vi "Start Module.vi"(6 "Show Main VI Diagram on Init (F)":bool, 8 "error in":errorcluster, 9 "Init Module ID":bool, 10 "Number of socket":i32, 11 "Run as Singleton? (F)":bool) -> (0 "error out":errorcluster, 1 "Wait for Event Sync?":bool, 2 "Test Unit Broadcast Events":T1, 3 "Module ID":i32)   [LabVIEW 2025, in "Test Unit.lvlib"]
doc: "Launches an instance of the module Main VI. After calling this VI, you can optionally register for broadcast events from the module by wiring the broadcast events output of this VI to a <b>Register For Events</b> function. \n\nAfter the optional Register For Events function call, you should always call the <b>Synchronize Module Events.vi</b> for this module with the 'Wait for Event Sync?' output of this VI to the corresponding input of the Synchronize Module Events.vi. \n\nTo see an example of the proper wiring pattern, see the \"Run New Module: Value Change\" event frame in the API Tester VI for this module.\n_____\nBased on DQMH Project Template 7.0.1.1316."
uses:
  Test Unit.lvlib
  Broadcast Events--cluster.ctl
  Did Init Argument--cluster.ctl
  Status Updated Argument--cluster.ctl
  Error Reported Argument--cluster.ctl
  Stop Argument--cluster.ctl
  Get Module Execution Status Argument--cluster.ctl
  Module Running State--enum.ctl
  <vilib>/Delacor/Delacor QMH/Libraries/Cloneable Module Admin_class/Delacor_lib_QMH_Cloneable Module Admin.lvclass
  C:/Program Files (x86)/National Instruments/LabVIEW 2025/vi.lib/Delacor/Delacor QMH/Libraries/Module Admin_class/Delacor_lib_QMH_Module Admin.lvclass
  VI Reference Management/Main VI Type--strict_vi_ref.ctl
  <vilib>/Delacor/Delacor QMH/Libraries/Cloneable Module Admin_class/Delacor_lib_QMH_Cloneable Module Admin.lvclass/Delacor_lib_QMH_Cloneable Module Admin.ctl
  <vilib>/Delacor/Delacor QMH/Libraries/Module Admin_class/Delacor_lib_QMH_Module Admin.lvclass/Delacor_lib_QMH_Module Admin.ctl
  <vilib>/Delacor/Delacor QMH/Libraries/Cloneable Module Admin_class/Delacor_lib_QMH_Set Module ID.vi
  <vilib>/Delacor/Delacor QMH/Libraries/Module Admin_class/Delacor_lib_QMH_Set External Launch.vi
  Clone Registration/Clone Registration.lvlib
  VI Reference Management/VI Reference Management.lvlib
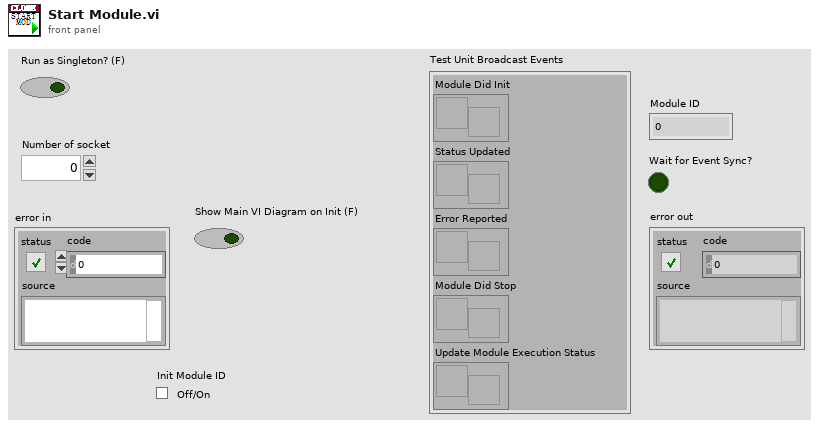
[diagram p1: front panel]
types:
  T1 = typedef "Test Unit.lvlib/Broadcast Events--cluster.ctl" = cluster{"Module Did Init":refnum<user-event>, "Status Updated":refnum<user-event>, "Error Reported":refnum<user-event>, "Module Did Stop":refnum<user-event>, "Update Module Execution Status":refnum<user-event>}
  T2 = typedef "Test Unit.lvlib/Module Running State--enum.ctl" = enum16{"Not Running", "Running as Cloneable", "Running as Singleton"}
  T3 = enum32{"Bad", "Idle", "Run top level", "Running"}
  T4 = typedef "Test Unit.lvlib/VI Reference Management.lvlib/Main VI Type--strict_vi_ref.ctl" = refnum<vi>
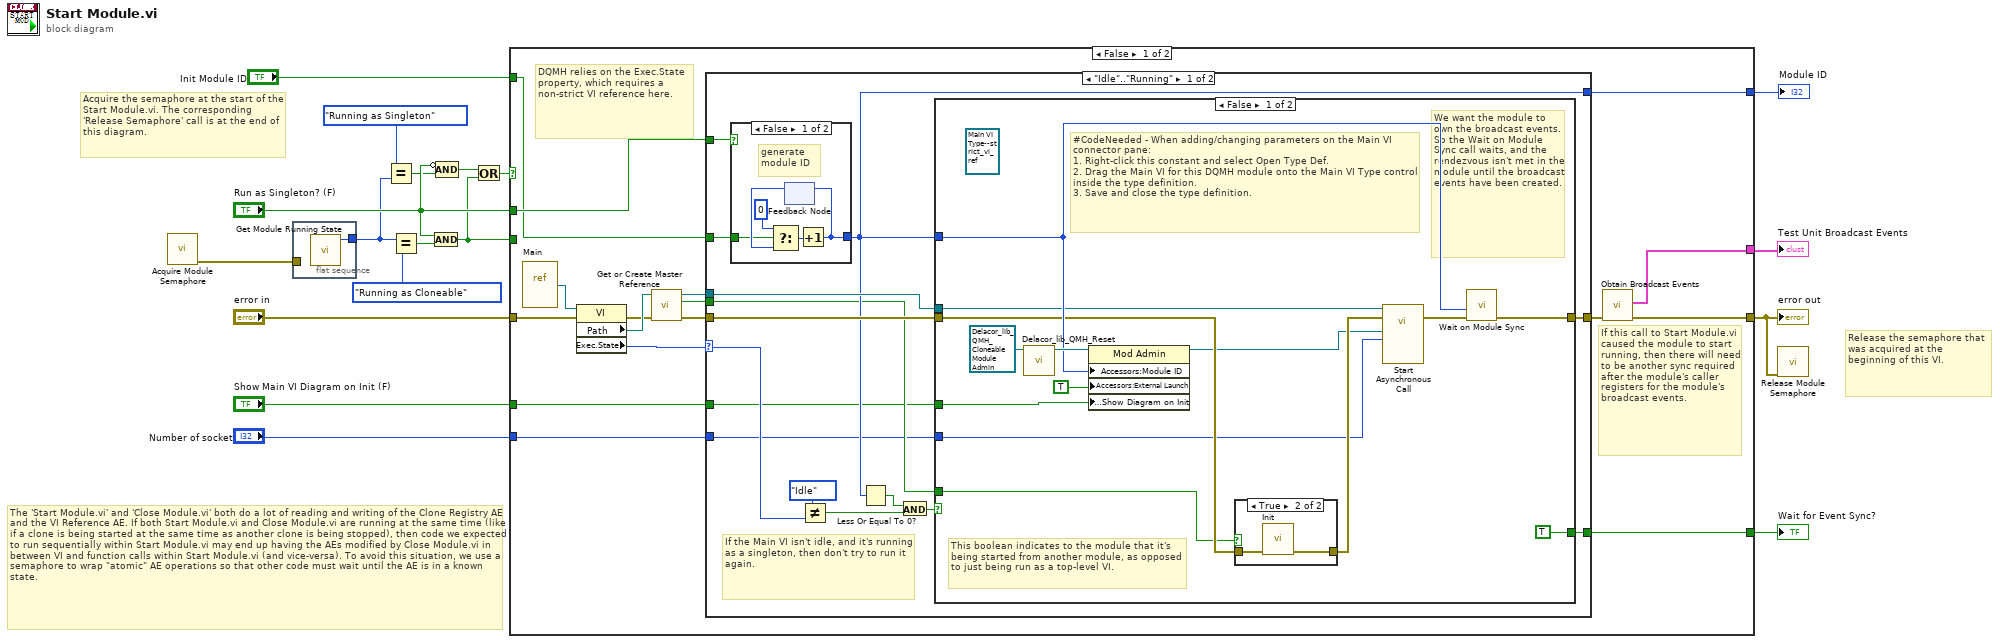
[diagram p0: block diagram]
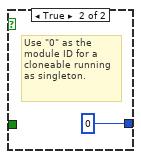
[diagram p2: hidden frame]
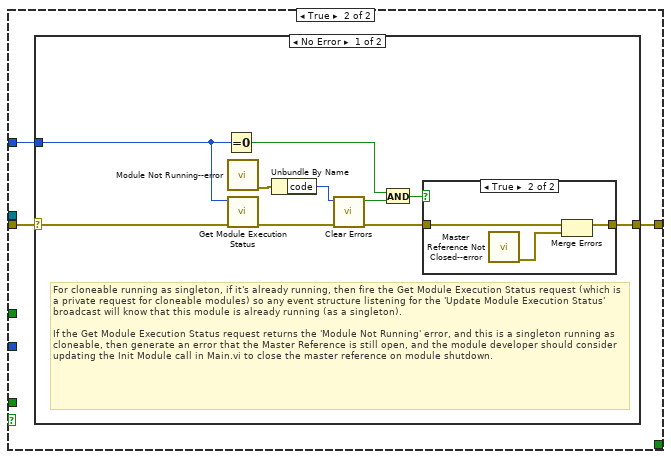
[diagram p4: hidden frame]
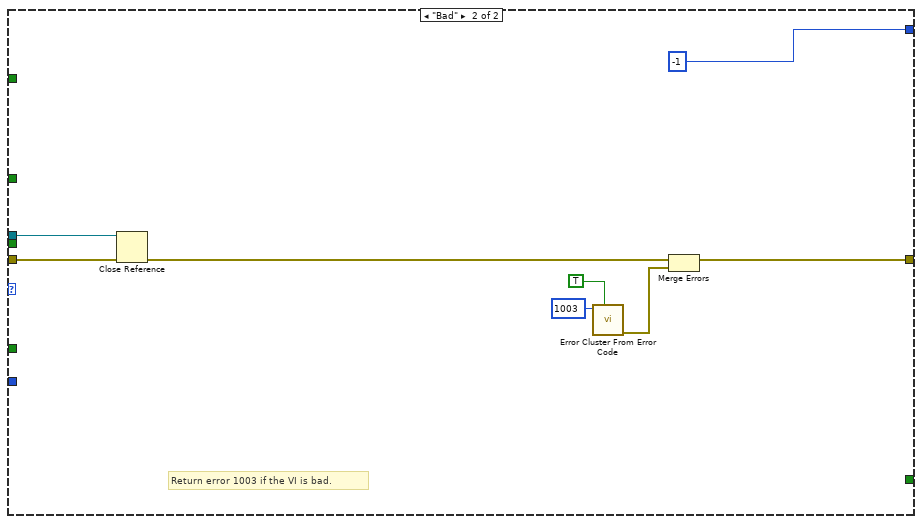
[diagram p7: hidden frame]
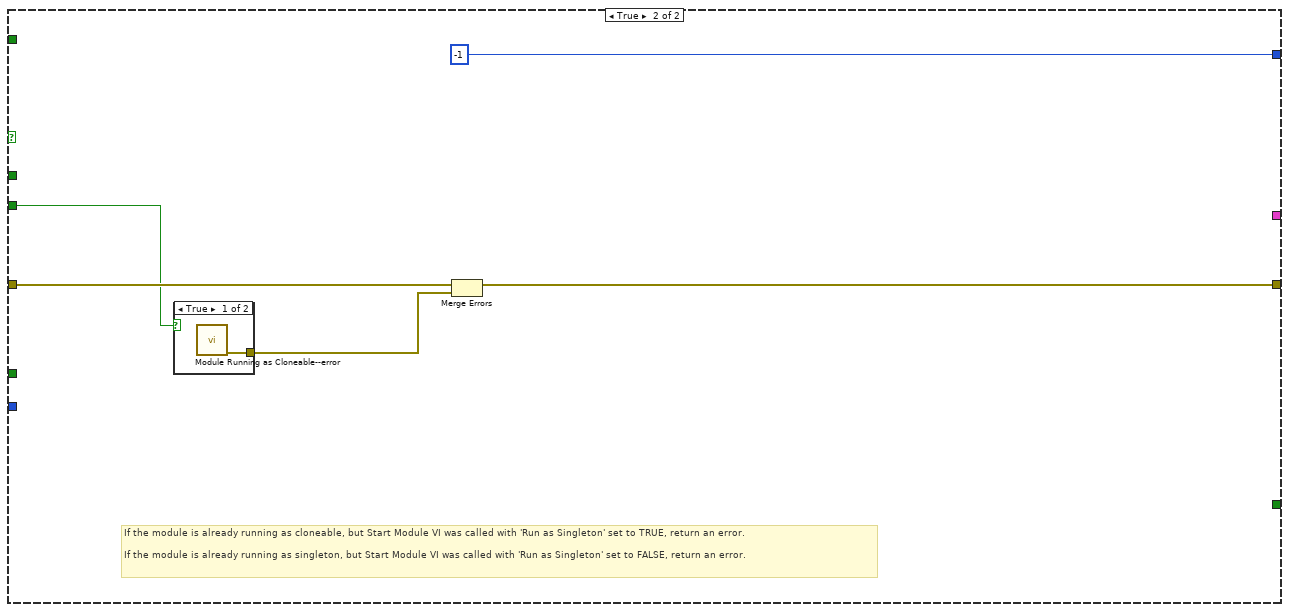
[diagram p8: hidden frame]
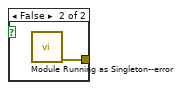
[diagram p9: hidden frame]
diagram:
  # "Release the semaphore that was acquired at the beginning of this VI."
  # "The 'Start Module.vi' and 'Close Module.vi' both do a lot of reading and writing of the Clone Registry AE and the VI Reference AE. If both Start Module.vi and Close Module.vi are running at the same time (like if a clone is being started at the same time as another clone is being stopped), then code we expected to run sequentially within Start Module.vi may end up having the AEs modified by Close Module.vi in between VI and function calls within Start Module.vi (and vice-versa). To avoid this situation, we use a semaphore to wrap \"atomic\" AE operations so that other code must wait until the AE is in a known state."
  # "Acquire the semaphore at the start of the Start Module.vi. The corresponding 'Release Semaphore' call is at the end of this diagram."
  n1 = call "Acquire Module Semaphore.vi"() -> ("error out"=w5:errorcluster)  [unwired: 11 in]
  n2 = flat-sequence {
    tunnel: [w19] -> w8
    tunnel: w5 -> [_]
    frame #0 {
      n3 = call "Get Module Running State.vi"() -> ("Module Running State"=w19:T2)  [unwired: 11 in]
    }
  }
  n4 = Equal?(x=Module_Running_State--enum."Running as Singleton", y=w8) -> (x = y?=w9:bool)
  n5 = Equal?(x=w8, y=Module_Running_State--enum."Running as Cloneable") -> (x = y?=w13:bool)
  n6 = And(x="Run as Singleton? (F)", y=w13) -> (x .and. y?=w6:bool)
  n7 = Compound Arithmetic op=AND(invert "Run as Singleton? (F)", w9) -> (w11:bool)
  n8 = Or(x=w11, y=w6) -> (x .or. y?=w12:bool)
  n9 = case shown="False" w12 {
    tunnel: "error in" -> [w36 w105]
    tunnel: [w34 w104] -> w4
    tunnel: [w33 _] -> w17
    tunnel: [w32 _] -> w16
    tunnel: [w28 -1] -> w15
    tunnel: "Run as Singleton? (F)" -> [w24 _]
    tunnel: w6 -> [_ w101]
    tunnel: "Show Main VI Diagram on Init (F)" -> [w22 _]
    tunnel: "Number of socket" -> [w21 _]
    tunnel: "Init Module ID" -> [w20 _]
    frame False {
      # "DQMH relies on the Exec.State property, which requires a non-strict VI reference here."
      # "If this call to Start Module.vi caused the module to start running, then there will need to be another sync required after the module's caller registers for the module's broadcast events."
      n10 = vi-ref "Main.vi"() -> (w27:refnum<vi>)
      n11 = property class="VI"(reference=w27, error in=w36) -> (error out=w30:errorcluster, "Path"=w31:path, "Exec.State"=w25:T3)  [unwired: 1 out]
      n12 = call "Get or Create Master Reference.vi"("error in"=w30, "Main VI Path"=w31) -> ("error out"=w29:errorcluster, "New Reference Created"=w23:bool, "Master Reference"=w26:T4)  [unwired: 7 in]
      n13 = case shown="\"Idle\"..\"Running\"" w25 {
        selector: w25 -> [w47 _]
        tunnel: w29 -> [w51 w100]
        tunnel: w26 -> [w49 w99]
        tunnel: [w48 w97] -> w35
        tunnel: [w50 _] -> w32
        tunnel: [w42 -1] -> w28
        tunnel: w24 -> [w41 _]
        tunnel: w23 -> [w40 _]
        tunnel: w22 -> [w39 _]
        tunnel: w21 -> [w38 _]
        tunnel: w20 -> [w37 _]
        frame "Idle".."Running" {
          # "If the Main VI isn't idle, and it's running as a singleton, then don't try to run it again."
          n14 = case shown="False" w41 {
            tunnel: [w56 0] -> w42
            tunnel: w37 -> [w52 _]
            frame False {
              # "generate module ID"
              n15 = feedback #1() -> (w54:i32)  [unwired: 1 in]
              n16 = Select(t=0, s=w52, f=w54) -> (s? t:f=w55:i32)
              n17 = Increment(x=w55) -> (x+1=w56:i32)
              n18 = feedback-in #1(w56) -> ()
            }
            frame True {
              # "Use \"0\" as the module ID for a cloneable running as singleton."
            }
          }
          n19 = Not Equal?(x=T3."Idle", y=w47) -> (x != y?=w45:bool)
          n20 = Less Or Equal To 0?(x=w42) -> (x <= 0?=w43:bool)
          n21 = And(x=w43, y=w45) -> (x .and. y?=w44:bool)
          n22 = case shown="False" w44 {
            tunnel: w51 -> [w63 w76]
            tunnel: [TRUE _] -> w50
            tunnel: w49 -> [w62 _]
            tunnel: [w66 w75] -> w48
            tunnel: w42 -> [w67 w77]
            tunnel: w40 -> [w60 _]
            tunnel: w39 -> [w59 _]
            tunnel: w38 -> [w58 _]
            frame False {
              (unwired) T4 refnum ("Main VI Type")
              # "#CodeNeeded - When adding/changing parameters on the Main VI connector pane:\n1. Right-click this constant and select Open Type Def.\n2. Drag the Main VI for this DQMH module onto the Main VI Type control inside the type definition.\n3. Save and close the type definition."
              # "We want the module to own the broadcast events. So the Wait on Module Sync call waits, and the rendezvous isn't met in the module until the broadcast events have been created."
              # "This boolean indicates to the module that it's being started from another module, as opposed to just being run as a top-level VI."
              n23 = call-dynamic "Delacor_lib_QMH_Reset.vi"("Mod Admin in"=refnum<class "Delacor_lib_QMH_Cloneable Module Admin.lvclass"> refnum) -> ("Mod Admin out"=w70:refnum<class "Delacor_lib_QMH_Cloneable Module Admin.lvclass">)  [unwired: 9 in, 1 out]
              n24 = property class="Mod Admin"(reference=w70, "Accessors:Module ID"=w67, "Accessors:External Launch"=TRUE, "Accessors:Show Diagram on Init"=w59) -> (reference out=w61:refnum<class "Delacor_lib_QMH_Cloneable Module Admin.lvclass">)  [unwired: 1 in, 1 out]
              n25 = case shown="True" w60 {
                tunnel: [w72 w74] -> w64
                tunnel: w63 -> [w72 w73]
                frame False {
                }
                frame True {
                  n26 = call "Init.vi"("error in"=w73) -> ("error out"=w74:errorcluster)  [unwired: 7 in, 3 out]
                }
              }
              n27 = call-by-ref "Start Asynchronous Call"(reference=w62, error in=w64, "Number of socket"=w58, "Module Admin"=w61) -> (error out=w65:errorcluster)  [unwired: 10 in, 1 out]
              n28 = call "Wait on Module Sync.vi"("error in"=w65, "Module ID"=w67) -> ("error out"=w66:errorcluster)  [unwired: 9 in]
            }
            frame True {
              n29 = case shown="No Error" w76 {
                selector: w76 -> [w87 w92]
                tunnel: w77 -> [w85 _]
                tunnel: [w78 w92] -> w75
                frame No Error {
                  # "For cloneable running as singleton, if it's already running, then fire the Get Module Execution Status request (which is a private request for cloneable modules) so any event structure listening for the 'Update Module Execution Status' broadcast will know that this module is already running (as a singleton).\n\nIf the Get Module Execution Status request returns the 'Module Not Running' error, and this is a singleton running as cloneable, then generate an error that the Master Reference is still open, and the module developer should consider updating the Init Module call in Main.vi to close the master reference on module shutdown."
                  n30 = Equal To 0?(x=w85) -> (x = 0?=w81:bool)
                  n31 = call "Module Not Running--error.vi"() -> ("error out"=w84:errorcluster)  [unwired: 11 in]
                  n32 = call "Get Module Execution Status.vi"("error in"=w87, "Module ID"=w85) -> ("error out"=w86:errorcluster)  [unwired: 9 in]
                  n33 = Unbundle By Name(w84) -> ("code"=w83:i32)
                  n34 = call <vilib>:"Clear Errors.vi"("error in (no error)"=w86, "specific error code to clear (0: all)"=w83) -> ("error out"=w80:errorcluster, "specific error cleared?"=w82:bool)  [unwired: 4 in]
                  n35 = And(x=w81, y=w82) -> (x .and. y?=w79:bool)
                  n36 = case shown="True" w79 {
                    tunnel: w80 -> [w88 w91]
                    tunnel: [w88 w89] -> w78
                    frame False {
                    }
                    frame True {
                      n37 = call "Master Reference Not Closed--error.vi"() -> ("error out"=w90:errorcluster)  [unwired: 11 in]
                      n38 = Merge Errors(w91, w90) -> (w89:errorcluster)
                    }
                  }
                }
                frame Error {
                }
              }
            }
          }
        }
        frame "Bad" {
          # "Return error 1003 if the VI is bad."
          n39 = Close Reference(reference=w99, error in (no error)=w100) -> (error out=w98:errorcluster)
          n40 = call <vilib>:"Error Cluster From Error Code.vi"("show call chain? (False)"=TRUE, "error code (0)"=1003) -> ("error out"=w95:errorcluster)  [unwired: 7 in]
          n41 = Merge Errors(w98, w95) -> (w97:errorcluster)
        }
      }
      n42 = call "Obtain Broadcast Events.vi"("error in"=w35) -> ("error out"=w34:errorcluster, "Test Unit Broadcast Events"=w33:T1)  [unwired: 9 in]
    }
    frame True {
      # "If the module is already running as cloneable, but Start Module VI was called with 'Run as Singleton' set to TRUE, return an error.\n\nIf the module is already running as singleton, but Start Module VI was called with 'Run as Singleton' set to FALSE, return an error."
      n43 = case shown="True" w101 {
        tunnel: [w106 w107] -> w102
        frame True {
          n44 = call "Module Running as Cloneable--error.vi"() -> ("error out"=w106:errorcluster)  [unwired: 11 in]
        }
        frame False {
          n45 = call "Module Running as Singleton--error.vi"() -> ("error out"=w107:errorcluster)  [unwired: 11 in]
        }
      }
      n46 = Merge Errors(w105, w102) -> (w104:errorcluster)
    }
  }
  "error out" <- w4
  "Test Unit Broadcast Events" <- w17
  "Wait for Event Sync?" <- w16
  "Module ID" <- w15
  n47 = call "Release Module Semaphore.vi"("error in"=w4) -> ()  [unwired: 10 in, 1 out]
